vi "Obtain Station Model.vi"(8 "error in (no error)":errorcluster, 11 "Engine in":refnum<class "Engine.lvclass">) -> (0 "error out":errorcluster, 2 "Station Model":refnum<class "SequenceFile.lvclass">, 3 "Engine out":refnum<class "Engine.lvclass">)   [LabVIEW 2020, in "TSnax.lvlib" / "Engine.lvclass"]
uses:
  Engine.lvclass
  Engine.lvclass/Engine.ctl
  PropertyObject/PropertyObject.lvclass
  SequenceFile/File Load Options.ctl
  SequenceFile/SequenceFile.lvclass
  C:/dev/illuminated-g/tsnax/TSnax/PropertyObjectFile/PropertyObjectFile.lvclass
  C:/dev/illuminated-g/tsnax/TSnax/PropertyObject/PropertyObject.lvclass
  C:/dev/illuminated-g/tsnax/TSnax/SequenceFile/SequenceFile.lvclass
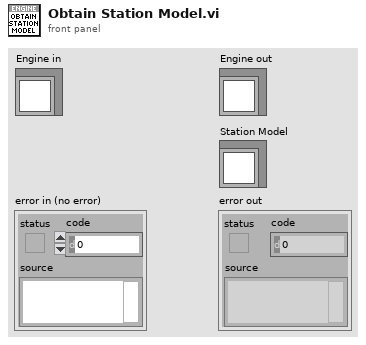
[diagram p1: front panel]
types:
  T1 = typedef "TSnax.lvlib/Engine.lvclass/Ref Data.ctl" = cluster{"Station Globals":refnum<class "PropertyObject.lvclass">, "Station Model":refnum<class "SequenceFile.lvclass">}
  T2 = typedef "TSnax.lvlib/SequenceFile.lvclass/File Load Options.ctl" = cluster{"Use Search Dirs? (T)":bool, "Conflict as Error? (T)":bool, "Check Station Model? (F)":bool, "Preload Modules? (T)":bool, "Skip Load Callback? (F)":bool, "Reload if Loaded? (F)":bool}
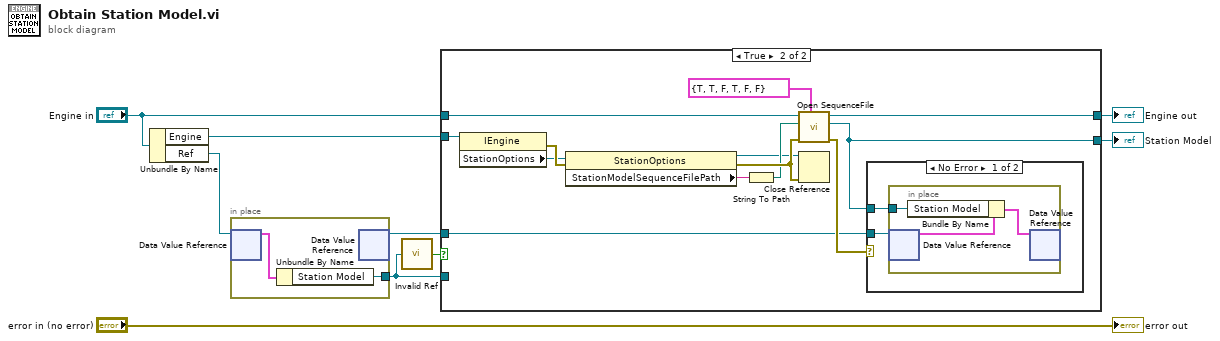
[diagram p0: block diagram]
diagram:
  n1 = Unbundle By Name("Engine in") -> ("Engine"=w4:refnum<k7>, "Ref"=w8:refnum<data-value>)
  n2 = in-place {
    in-place-border: [w10] -> w6
    n3 = in-place-dvr #1(w8) -> (w11:T1)  [unwired: 1 out]
    n4 = Unbundle By Name(w11) -> ("Station Model"=w10:refnum<class "SequenceFile.lvclass">)
    n5 = in-place-dvr #1() -> (w1:refnum<data-value>)  [unwired: 1 in, 1 out]
  }
  n6 = call "Invalid Ref.vi"("PropertyObject"=w6) -> ("Not a Valid Ref?"=w7:bool)
  n7 = case shown="True" w7 {
    tunnel: w6 -> [w13 _]
    tunnel: [w13 w15] -> w5
    tunnel: w4 -> [_ w20]
    tunnel: "Engine in" -> [w12 w25]
    tunnel: [w12 w17] -> w2
    tunnel: w1 -> [_ w14]
    frame False {
    }
    frame True {
      n8 = property class="IEngine"(reference=w20) -> (error out=w23:errorcluster, "StationOptions"=w22:refnum<k7>)  [unwired: 1 in, 1 out]
      n9 = property class="StationOptions"(reference=w22, error in=w23) -> (reference out=w18:refnum<k7>, error out=w26:errorcluster, "StationModelSequenceFilePath"=w21:string)
      n10 = String To Path(string=w21) -> (path=w19:path)
      n11 = call "Open SequenceFile.vi"("File Load Options"=T2 {"Use Search Dirs? (T)"=TRUE, "Conflict as Error? (T)"=TRUE, "Check Station Model? (F)"=FALSE, "Preload Modules? (T)"=TRUE, "Skip Load Callback? (F)"=FALSE, "Reload if Loaded? (F)"=FALSE}, "error in (no error)"=w26, "File Path"=w19, "Engine in"=w25) -> ("error out"=w16:errorcluster, "SequenceFile"=w15:refnum<class "SequenceFile.lvclass">, "Engine out"=w17:refnum<class "Engine.lvclass">)  [unwired: 5 in]
      n12 = Close Reference(reference=w18, error in (no error)=w26) -> ()  [unwired: 1 out]
      n13 = case shown="No Error" w16 {
        tunnel: w15 -> [w27 _]
        tunnel: w14 -> [w28 _]
        frame No Error {
          n14 = in-place {
            in-place-border: w27 -> [w30]
            n15 = in-place-dvr #2(w28) -> (w31:T1)  [unwired: 1 out]
            n16 = Bundle By Name(cluster=w31, "Station Model"=w30) -> (w29:T1)
            n17 = in-place-dvr #2(w29) -> ()  [unwired: 2 out]
          }
        }
        frame Error {
        }
      }
    }
  }
  "Engine out" <- w2
  "Station Model" <- w5
  "error out" <- "error in (no error)"
